vi "Set.vi"(8 "error in (no error)":errorcluster, 10 "Data":variant, 11 "AbstractData in":refnum<class "AbstractData.lvclass">) -> (0 "error out":errorcluster, 3 "AbstractData out":refnum<class "AbstractData.lvclass">)   [LabVIEW 2014, in "AbstractData.lvclass"]
uses:
  AbstractData.lvclass
  AbstractData.lvclass/AbstractData.ctl
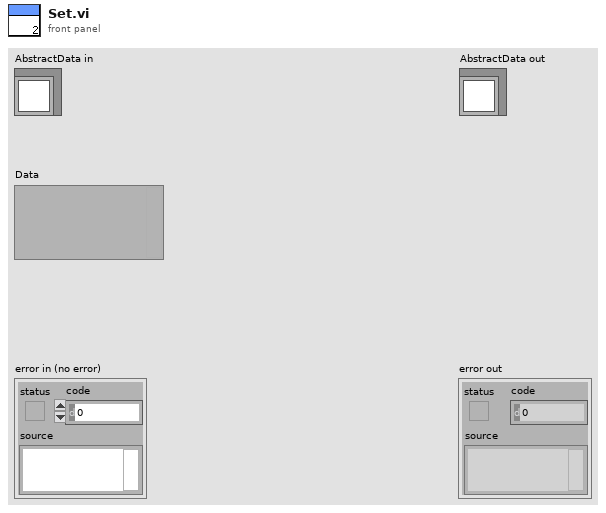
[diagram p1: front panel]
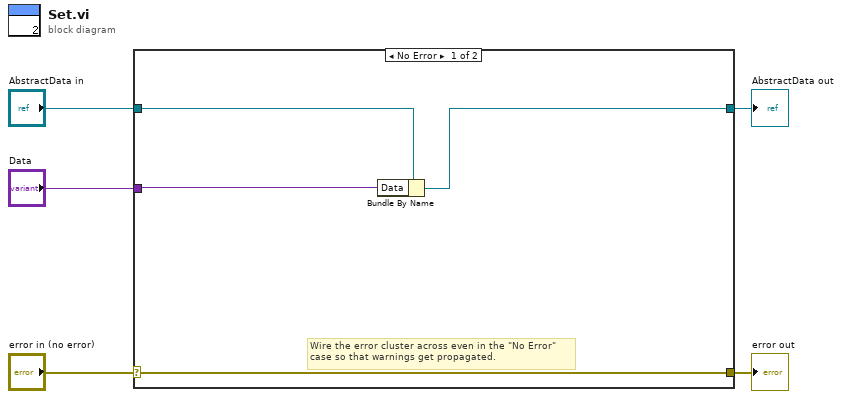
[diagram p0: block diagram]
diagram:
  n1 = case shown="No Error" "error in (no error)" {
    selector: "error in (no error)" -> [w9 w11]
    tunnel: [w9 w11] -> w4
    tunnel: [w7 w10] -> w2
    tunnel: "AbstractData in" -> [w8 w10]
    tunnel: "Data" -> [w6 _]
    frame No Error {
      # "Wire the error cluster across even in the \"No Error\"\ncase so that warnings get propagated."
      n2 = Bundle By Name(cluster=w8, "Data"=w6) -> (w7:refnum<class "AbstractData.lvclass">)
    }
    frame Error {
    }
  }
  "error out" <- w4
  "AbstractData out" <- w2
